vi "ReplaceOutsideItems.vi"(8 "error in (no error)":errorcluster, 9 "Project:Open":refnum<vi>, 10 "OutsideVIs":string[](array[string]), 11 "DestinationDirectory":path) -> (0 "error out":errorcluster)   [LabVIEW 2021, in "Migrator.lvlib"]
uses:
  Migrator.lvlib
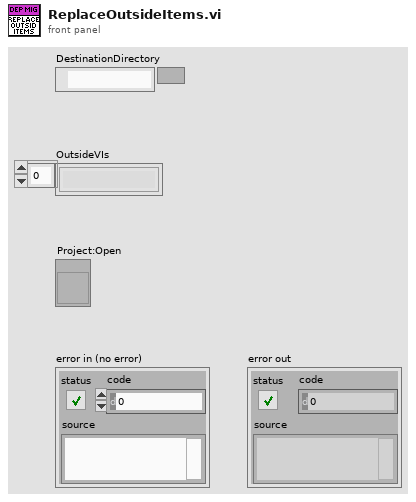
[diagram p1: front panel]
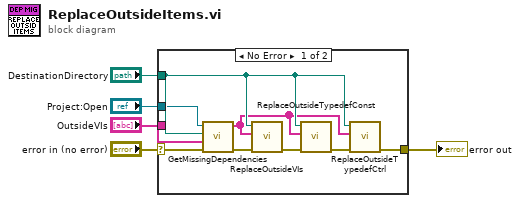
[diagram p0: block diagram]
diagram:
  n1 = case shown="No Error" "error in (no error)" {
    selector: "error in (no error)" -> [w6 w15]
    tunnel: "OutsideVIs" -> [w14 _]
    tunnel: [w13 w15] -> w4
    tunnel: "DestinationDirectory" -> [w10 _]
    tunnel: "Project:Open" -> [w7 _]
    frame No Error {
      n2 = call "GetMissingDependencies.vi"("error in (no error)"=w6, "OutsideVIs in"=w14, "DestinationDirectory"=w10, "Project in"=w7) -> ("error out"=w9:errorcluster, "OutsideVIs out"=w8:string[])  [unwired: 6 in]
      n3 = call "ReplaceOutsideVIs.vi"("error in (no error)"=w9, "Non-Library VI[]"=w8, "TargetDirectory"=w10) -> ("error out"=w11:errorcluster)  [unwired: 8 in]
      n4 = call "ReplaceOutsideTypedefConst.vi"("error in (no error)"=w11, "Non-Library VI[]"=w8, "TargetDirectory"=w10) -> ("error out"=w12:errorcluster)  [unwired: 8 in]
      n5 = call "ReplaceOutsideTypedefCtrl.vi"("error in (no error)"=w12, "Non-Library VI[]"=w8, "TargetDirectory"=w10) -> ("error out"=w13:errorcluster)  [unwired: 8 in]
    }
    frame Error {
    }
  }
  "error out" <- w4
